vi "Query User.vi"(0 "VISA resource name":refnum<visa-resource-name>, 5 "User Pointer(0-299)":i32=1, 11 "error in (no error)":errorcluster) -> (4 "VISA resource name out":refnum<visa-resource-name>, 6 "User Name (8 character max)":string, 8 "Password (8 number max)":string, 10 "Level":u16(ring)=1 items=["Run Only", "Recall Setup", "Edit Step", "Full System"], 15 "error out":errorcluster)   [LabVIEW 2020, in "eec EST 300.lvlib"]
doc: "Query the User setting.\n1.User Pointer\n2.User ID\n3.Password\n4.Security Level:\n 0=Run Only, This is the most restricted mode of user access. You can only initiate a test, reset a failure or abort a test from the Perform Tests screen.\n\n 1=Recall Setup, This mode allows you to load previously configured test files but it does not allow any editing of the parameters. In this mode you are restricted from access to the “Setup Test Parameters” screen.\n\n 2=Edit Step, In this mode you can load files and edit test parameters.\n\n 3=Full System, In this mode you have full access level to all instrument setup parameters as well as system configuration and security levels. Access at this level should be restricted to System Administrators."
uses:
  <instrlib>/eec EST 300/eec EST 300.lvlib
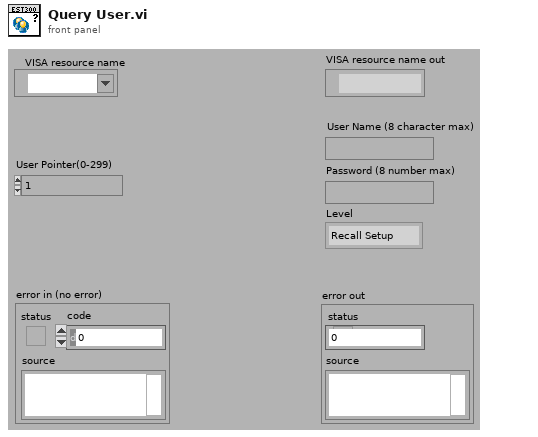
[diagram p1: front panel]
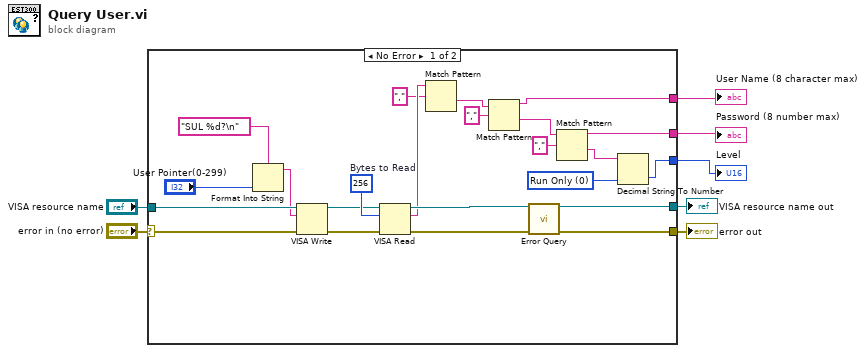
[diagram p0: block diagram]
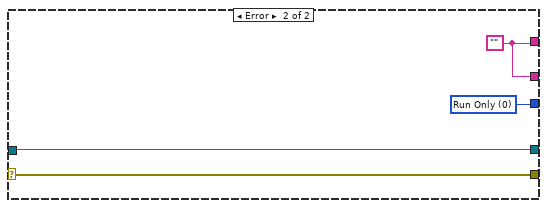
[diagram p2: hidden frame]
diagram:
  n1 = case shown="No Error" "error in (no error)" {
    selector: "error in (no error)" -> [w30 w34]
    tunnel: [w13 w34] -> w4
    tunnel: [w12 w33] -> w5
    tunnel: "VISA resource name" -> [w29 w33]
    tunnel: [w19 w31] -> w1
    tunnel: [w24 w32] -> w3
    tunnel: [w22 w32] -> w2
    frame No Error {
      w18 = u16 0 items=["Run Only", "Recall Setup", "Edit Step", "Full System"] ("Level")
      w28 = u32 256  # Bytes to Read
      n2 = Format Into String(format string="SUL %d?\n" ("Command to Send (empty)"), "User Pointer(0-299)") -> (resulting string=w16:string)  [unwired: 2 in, 1 out]
      n3 = VISA Write(VISA resource name=w29, write buffer=w16, error in (no error)=w30) -> (VISA resource name out=w27:refnum<visa-resource-name>, error out=w26:errorcluster)  [unwired: 1 out]
      n4 = VISA Read(VISA resource name=w27, byte count=w28, error in (no error)=w26) -> (VISA resource name out=w11:refnum<visa-resource-name>, read buffer=w10:string, error out=w14:errorcluster)  [unwired: 1 out]
      n5 = Match Pattern(string=w10, regular expression=",") -> (after substring=w9:string)  [unwired: 1 in, 3 out]
      n6 = Match Pattern(string=w9, regular expression=",") -> (before substring=w24:string, after substring=w23:string)  [unwired: 1 in, 2 out]
      n7 = call <instrlib>:"Error Query.vi"("VISA resource name"=w11, "error in (no error)"=w14) -> ("VISA resource name out"=w12:refnum<visa-resource-name>, "error out"=w13:errorcluster)  [unwired: 10 in, 2 out]
      n8 = Match Pattern(string=w23, regular expression=",") -> (before substring=w22:string, after substring=w20:string)  [unwired: 1 in, 2 out]
      n9 = Decimal String To Number(string=w20, default (0L)=w18) -> (number=w19:u16)  [unwired: 1 in, 1 out]
    }
    frame Error {
      w31 = u16 0 items=["Run Only", "Recall Setup", "Edit Step", "Full System"] ("Level")
      w32 = ""
    }
  }
  "VISA resource name out" <- w5
  "error out" <- w4
  "Password (8 number max)" <- w2
  "User Name (8 character max)" <- w3
  "Level" <- w1
